vi "DBL.vi"(4 "Value":dbl) -> (1 "Constant":refnum<class "Const_DBL.lvclass">)   [LabVIEW 2021, in "Const_DBL.lvclass"]
uses:
  Const_DBL.lvclass
  Const_DBL.lvclass/Const_DBL.ctl
  Properties/Write Value.vi
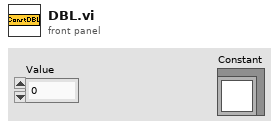
[diagram p1: front panel]
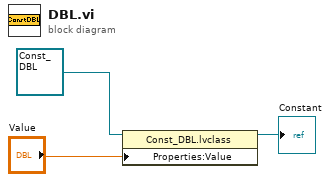
[diagram p0: block diagram]
diagram:
  n1 = property class="Const_DBL.lvclass"(reference=refnum<class "Const_DBL.lvclass"> refnum ("Constants.lvlib:Numeric.lvclass"), "Properties:Value"="Value") -> (reference out=→"Constant":refnum<class "Const_DBL.lvclass">)  [unwired: 1 in, 1 out]
